vi "FT10_Semi-Auto Set Mode.vi"(7 "Wait Time (ms)":i32=10, 9 "Mode in":T2, 10 "Port in":T1) -> (1 "Mode out":T2, 2 "Port out":T1, 3 "Command Cluster":T3)   [LabVIEW 2024]
doc: "Creates message for Message Handling Loop to set mode on port for the upcoming activation."
uses:
  Controls/Control_Command Cluster.ctl
  Controls/Control_Semi-Auto Port.ctl
  Controls/Control_Semi-Auto Mode.ctl
  Controls/Control_Fornax Mono1 Cut Enum.ctl
  Controls/Control_Fornax Mono1 Coag Enum.ctl
  Controls/Control_Fornax Mono2 Cut Enum.ctl
  Controls/Control_Fornax Mono2 Coag Enum.ctl
  Controls/Control_Fornax Bipolar Enum.ctl
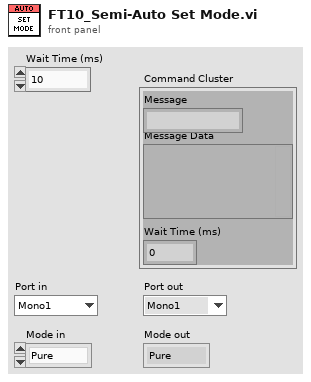
[diagram p1: front panel]
types:
  T1 = typedef "Control_Semi-Auto Port.ctl" = enum16{"Mono1", "Mono2", "Bipolar", "Ligasure", "Error"}
  T2 = typedef "Control_Semi-Auto Mode.ctl" = enum16{"Pure", "Blend", "Spray", "Fulgerate", "Standard", "Macro", "Precision", "Ligasure", "Error"}
  T3 = typedef "Control_Command Cluster.ctl" = cluster{"Message":string, "Message Data":variant, "Wait Time (ms)":i32}
  T4 = typedef "Control_Fornax Mono1 Cut Enum.ctl" = enum16{"Pure", "Blend"}
  T5 = typedef "Control_Fornax Mono1 Coag Enum.ctl" = enum16{"Fulgerate", "Spray"}
  T6 = typedef "Control_Fornax Mono2 Cut Enum.ctl" = enum16{"Pure", "Blend"}
  T7 = typedef "Control_Fornax Mono2 Coag Enum.ctl" = enum16{"Fulgerate", "Spray"}
  T8 = typedef "Control_Fornax Bipolar Enum.ctl" = enum16{"Standard", "Macro", "Precision"}
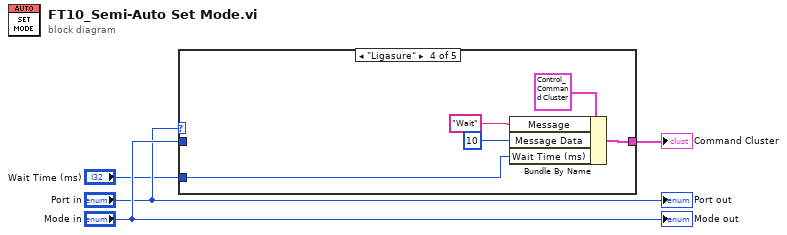
[diagram p0: block diagram]
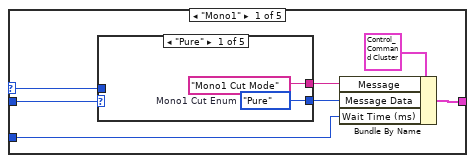
[diagram p2: hidden frame]
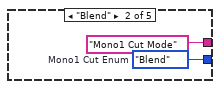
[diagram p3: hidden frame]
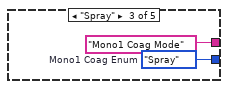
[diagram p4: hidden frame]
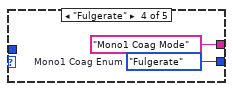
[diagram p5: hidden frame]
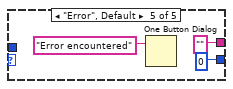
[diagram p6: hidden frame]
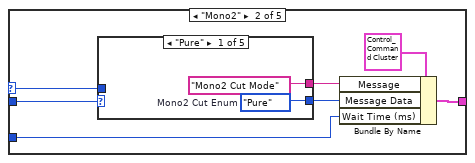
[diagram p7: hidden frame]
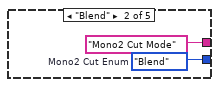
[diagram p8: hidden frame]
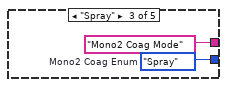
[diagram p9: hidden frame]
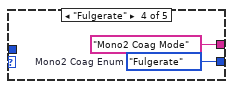
[diagram p10: hidden frame]
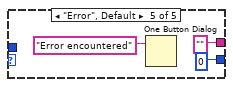
[diagram p11: hidden frame]
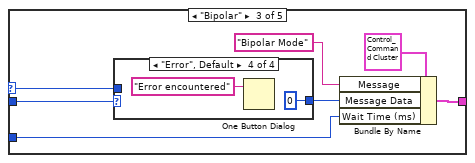
[diagram p12: hidden frame]
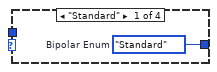
[diagram p13: hidden frame]
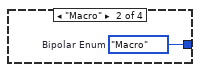
[diagram p14: hidden frame]
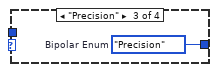
[diagram p15: hidden frame]
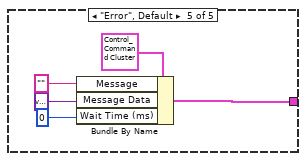
[diagram p16: hidden frame]
diagram:
  n1 = case shown="\"Ligasure\"" "Port in" {
    selector: "Port in" -> [w7 w25 w43 _ _]
    tunnel: "Mode in" -> [w6 w24 w42 _ _]
    tunnel: [w8 w26 w44 w55 w58] -> w2
    tunnel: "Wait Time (ms)" -> [w5 w23 w41 w53 _]
    frame "Mono1" {
      n2 = case shown="\"Pure\"" w6 {
        tunnel: w7 -> [_ _ _ _ _]
        tunnel: [w12 w14 w16 w18 u16 0 ("Mono2 Coag Enum")] -> w9
        tunnel: ["Mono1 Cut Mode" ("Message") "Mono1 Cut Mode" ("Message") "Mono1 Coag Mode" ("Message") "Mono1 Coag Mode" ("Message") "" ("Message")] -> w10
        frame "Pure" {
          w12 = Control_Fornax_Mono1_Cut_Enum."Pure"  # Mono1 Cut Enum
        }
        frame "Blend" {
          w14 = Control_Fornax_Mono1_Cut_Enum."Blend"  # Mono1 Cut Enum
        }
        frame "Spray" {
          w16 = Control_Fornax_Mono1_Coag_Enum."Spray"  # Mono1 Coag Enum
        }
        frame "Fulgerate" {
          w18 = Control_Fornax_Mono1_Coag_Enum."Fulgerate"  # Mono1 Coag Enum
        }
        frame "Error", Default {
          n3 = One Button Dialog(message="Error encountered") -> ()  [unwired: 1 in, 1 out]
        }
      }
      n4 = Bundle By Name(cluster=T3 {"Message"="", "Message Data"=variant, "Wait Time (ms)"=0}, "Message"=w10, "Message Data"=w9, "Wait Time (ms)"=w5) -> (w8:T3)
    }
    frame "Mono2" {
      n5 = case shown="\"Pure\"" w24 {
        tunnel: w25 -> [_ _ _ _ _]
        tunnel: [w31 w33 w35 w37 u16 0 ("Mono2 Coag Enum")] -> w27
        tunnel: ["Mono2 Cut Mode" ("Message") "Mono2 Cut Mode" ("Message") "Mono2 Coag Mode" ("Message") "Mono2 Coag Mode" ("Message") "" ("Message")] -> w28
        frame "Pure" {
          w31 = Control_Fornax_Mono2_Cut_Enum."Pure"  # Mono2 Cut Enum
        }
        frame "Blend" {
          w33 = Control_Fornax_Mono2_Cut_Enum."Blend"  # Mono2 Cut Enum
        }
        frame "Spray" {
          w35 = Control_Fornax_Mono2_Coag_Enum."Spray"  # Mono2 Coag Enum
        }
        frame "Fulgerate" {
          w37 = Control_Fornax_Mono2_Coag_Enum."Fulgerate"  # Mono2 Coag Enum
        }
        frame "Error", Default {
          n6 = One Button Dialog(message="Error encountered") -> ()  [unwired: 1 in, 1 out]
        }
      }
      n7 = Bundle By Name(cluster=T3 {"Message"="", "Message Data"=variant, "Wait Time (ms)"=0}, "Message"=w28, "Message Data"=w27, "Wait Time (ms)"=w23) -> (w26:T3)
    }
    frame "Bipolar" {
      n8 = case shown="\"Error\", Default" w42 {
        tunnel: w43 -> [_ _ _ _]
        tunnel: [w48 w49 w50 u16 0 ("Mono2 Coag Enum")] -> w45
        frame "Standard" {
          w48 = Control_Fornax_Bipolar_Enum."Standard"  # Bipolar Enum
        }
        frame "Macro" {
          w49 = Control_Fornax_Bipolar_Enum."Macro"  # Bipolar Enum
        }
        frame "Precision" {
          w50 = Control_Fornax_Bipolar_Enum."Precision"  # Bipolar Enum
        }
        frame "Error", Default {
          n9 = One Button Dialog(message="Error encountered") -> ()  [unwired: 1 in, 1 out]
        }
      }
      n10 = Bundle By Name(cluster=T3 {"Message"="", "Message Data"=variant, "Wait Time (ms)"=0}, "Message"="Bipolar Mode", "Message Data"=w45, "Wait Time (ms)"=w41) -> (w44:T3)
    }
    frame "Ligasure" {
      n11 = Bundle By Name(cluster=T3 {"Message"="", "Message Data"=variant, "Wait Time (ms)"=0}, "Message"="Wait", "Message Data"=10 ("Wait Time (ms)"), "Wait Time (ms)"=w53) -> (w55:T3)
    }
    frame "Error", Default {
      n12 = Bundle By Name(cluster=T3 {"Message"="", "Message Data"=variant, "Wait Time (ms)"=0}, "Message"="", "Message Data"=variant, "Wait Time (ms)"=0) -> (w58:T3)
    }
  }
  "Command Cluster" <- w2
  "Port out" <- "Port in"
  "Mode out" <- "Mode in"
